vi "read from Volt Meter.vi"(1 "Address":string="24") -> (0 "Data":string)   [LabVIEW 2012]
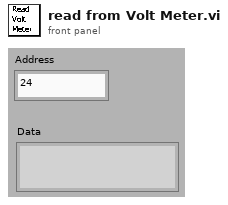
[diagram p1: front panel]
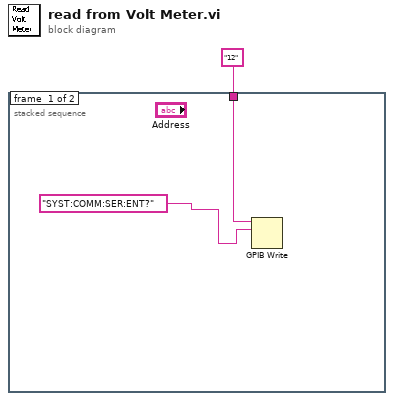
[diagram p0: block diagram]
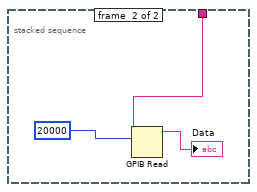
[diagram p2: hidden frame]
diagram:
  n1 = stacked-sequence {
    tunnel: "12" ("address string") -> [w2 w6]
    frame #0 {
      n2 = GPIB Write(0:w2, 1:"SYST:COMM:SER:ENT?" ("string")) -> ()  [unwired: 3 in, 2 out]
    }
    frame #1 {
      n3 = GPIB Read(0:w6, 1:20000 ("byte count")) -> (5:→"Data":string)  [unwired: 3 in, 2 out]
    }
  }
